vi "Responder.vi"() -> ()   [LabVIEW 2024]
uses:
  src/NATS Subscription/NATS Subscription.lvclass/NATS Subscription.ctl
  src/NATS Client/NATS Client.lvclass/NATS Client.ctl
  src/NATS Subscription/NATS Subscription.lvclass
  src/NATS Client/NATS Client.lvclass
panel:
  out "error out":errorcluster
  # "Run this VI then run Requester.vi.\n\nThis VI will repond to requests."
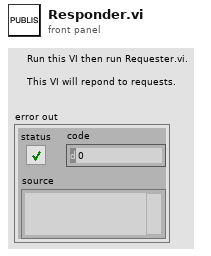
[diagram p1: front panel]
types:
  T1 = typedef "NATS Core.lvlib/nats message.ctl" = cluster{"subject":string, "payload":string, "sub id":string, "reply-to":string, "headers":string, "type":T2, "received":timestamp}
  T2 = typedef "NATS Core.lvlib/msg type.ctl" = enum16{"Undefined", "MSG", "HMSG", "+OK", "PING", "PONG", "-ERR", "INFO"}
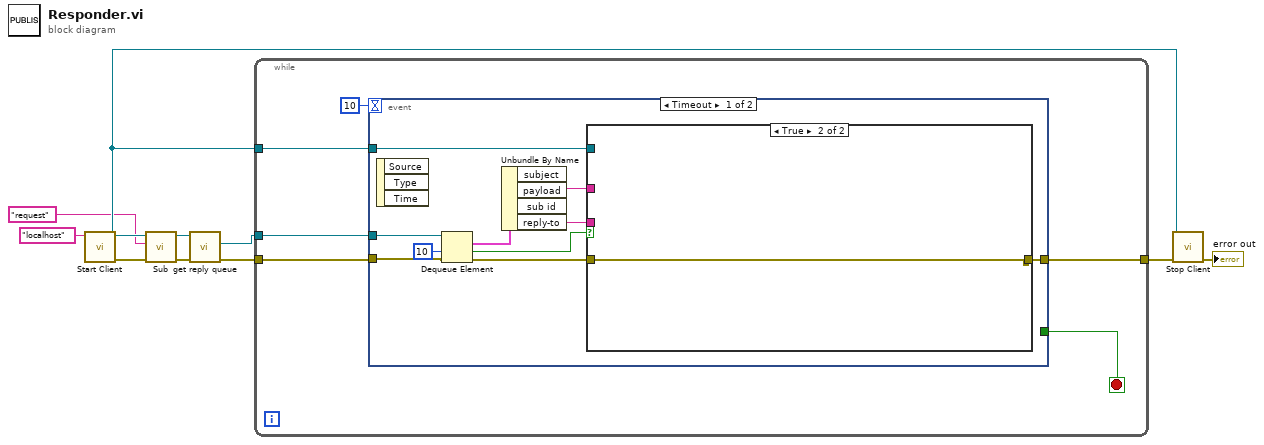
[diagram p0: block diagram]
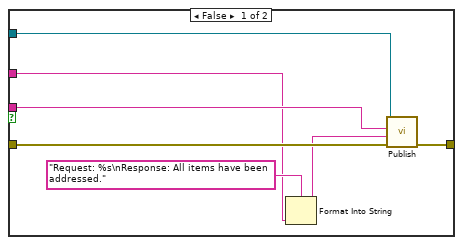
[diagram p2: hidden frame]
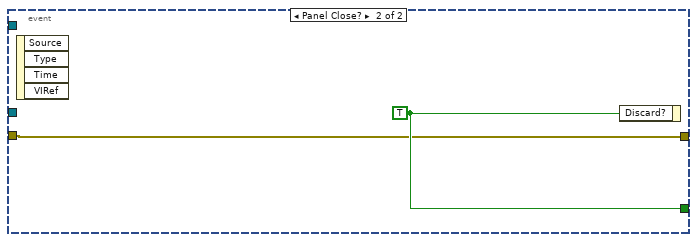
[diagram p3: hidden frame]
diagram:
  n1 = call "Start Client.vi"("address"="localhost") -> ("error out"=w6:errorcluster, "NATS Client out"=w7:refnum<class "NATS Client.lvclass">)  [unwired: 9 in]
  n2 = call "Sub.vi"("error in"=w6, "subject"="request" ("Request Subject"), "NATS Client"=w7) -> ("error out"=w1:errorcluster, "NATS Subscription"=w5:refnum<class "NATS Subscription.lvclass">)  [unwired: 7 in]
  n3 = call "get reply queue.vi"("error in"=w1, "NATS Subscription in"=w5) -> ("error out"=w4:errorcluster, "reply queue"=w3:refnum<queue>)  [unwired: 7 in, 1 out]
  n4 = while {
    tunnel: w7 -> [w16]
    tunnel: [w15] -> w9
    tunnel: w4 -> [w13]
    tunnel: w3 -> [w12]
    stop <- w11 stop-if-true
    n5 = event shown="[0] Timeout" {
      selector: _ -> [_ _]
      dyn-events: _ -> [_ _]
      timeout: 10 -> [_ _]
      tunnel: w13 -> [w26 w35]
      tunnel: w16 -> [w25 _]
      tunnel: [w20 w35] -> w15
      tunnel: w12 -> [w19 _]
      tunnel: [_ w36] -> w11
      event Timeout {
        n6 = event-data() -> ()  [unwired: 1 in, 3 out]
        n7 = Dequeue Element(queue=w19, timeout in ms (-1)=10, error in (no error)=w26) -> (element=w23:T1, timed out?=w17:bool, error out=w24:errorcluster)  [unwired: 1 out]
        n8 = Unbundle By Name(w23) -> ("payload"=w21:string, "reply-to"=w22:string)  [unwired: 2 out]
        n9 = case shown="True" w17 {
          tunnel: w25 -> [w33 _]
          tunnel: w24 -> [w32 w34]
          tunnel: w22 -> [w31 _]
          tunnel: w21 -> [w29 _]
          tunnel: [w27 w34] -> w20
          frame False {
            n10 = Format Into String(format string="Request: %s\nResponse: All items have been addressed.", w29) -> (resulting string=w28:string)  [unwired: 2 in, 1 out]
            n11 = call "Publish.vi"("error in"=w32, "payload"=w28, "subject"=w31, "NATS Client.lvlib:NATS Client.lvclass"=w33) -> ("error out"=w27:errorcluster)  [unwired: 7 in]
          }
          frame True {
          }
        }
      }
      event Panel Close? {
        w36 = TRUE ("Discard?")
        n12 = event-data() -> ()  [unwired: 1 in, 4 out]
        n13 = event-data("Discard?"=w36) -> ()  [unwired: 1 in, 1 out]
      }
    }
  }
  n14 = call "Stop Client.vi"("error in"=w9, "NATS Client"=w7) -> ("error out"=→"error out":errorcluster)  [unwired: 9 in]
